vi "Target.vi"(4 "Refnums":T3, 7 "Images":T2[](array[typedef]), 8 "error in (no error)":errorcluster, 10 "Pattern Matching Criteria":T4={"Minimum Score"=700.0, "Color Score Weight"=700.0, "Minimum Contrast"=50, "Match Mode"=0, "Match Feature Mode"=0, "Subpixel Accuracy"=TRUE, "Color Sensitivity"=1, "Search Strategy"=1} {"Search Strategy" items=["Conservative", "Balance", "Aggressive", "Very Aggressive"]; "Color Sensitivity" items=["Low Sensitivity", "Medium Sensitivity", "High Sensitivity"]; "Match Feature Mode" items=["Color and Shape", "Color", "Shape"]; "Match Mode" items=["Shift Invariant", "Rotation Invariant"]}, 11 "Function":T5) -> (0 "error out":errorcluster, 2 "Target Data":T1, 3 "Target Found?":bool)   [LabVIEW 2014]
uses:
  Target Functions.ctl
  Target Refnums.ctl
  <vilib>/vision/Image Controls.llb/IMAQ Image.ctl
  <vilib>/vision/NI_Vision_Development_Module.lvlib
panel:
  out "Edge":T2(plugin-control)
  out "Image":T2(plugin-control)
  out "Template":T2(plugin-control)
  # "LICENSED MATERIALS – PROPERTY OF IBM\nCopyright IBM Corp. 2016,\nALL RIGHTS RESERVED"
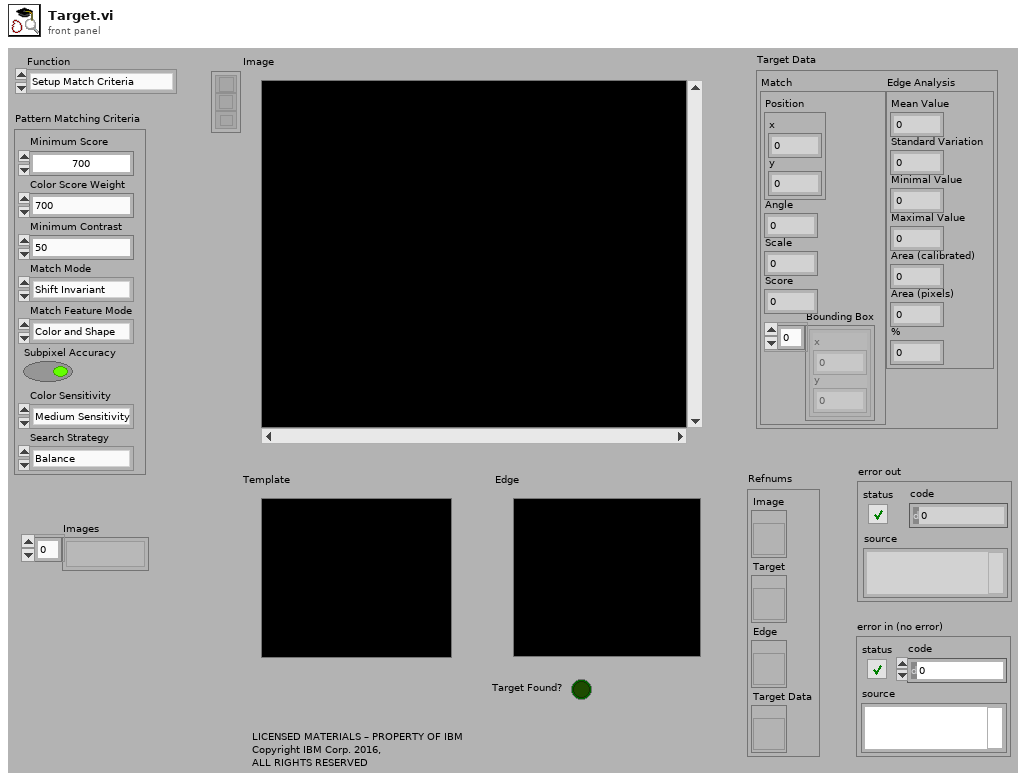
[diagram p1: front panel]
types:
  T1 = cluster{"Match":cluster{"Position":cluster{"x":sgl, "y":sgl}, "Angle":sgl, "Scale":sgl, "Score":sgl, "Bounding Box":cluster{"x":sgl, "y":sgl}[]}, "Edge Analysis":cluster{"Mean Value":sgl, "Standard Variation":sgl, "Minimal Value":sgl, "Maximal Value":sgl, "Area (calibrated)":sgl, "Area (pixels)":i32, "%":sgl}}
  T2 = typedef "IMAQ Image.ctl" = refnum<image>
  T3 = typedef "Target Refnums.ctl" = cluster{"Image":refnum<vi>, "Target":refnum<vi>, "Edge":refnum<vi>, "Target Data":refnum<vi>}
  T4 = cluster{"Minimum Score":sgl, "Color Score Weight":sgl, "Minimum Contrast":i32, "Match Mode":u32, "Match Feature Mode":u32, "Subpixel Accuracy":bool, "Color Sensitivity":u32, "Search Strategy":u32}
  T5 = typedef "Target Functions.ctl" = enum16{"Setup Match Criteria", "Set Target", "Find Target"}
  T6 = enum32{"Differentiation", "Gradient", "Prewitt", "Roberts", "Sigma", "Sobel"}
  T7 = cluster{i32[], cluster{"Contour Type":u32, "ROI Type":u32, i32[]}[]}
  T8 = cluster{"Global Rectangle":i32[], "Contours":cluster{"Contour Type":u32, "ROI Type":u32, "Points":i32[]}[]}
  T9 = cluster{"Position":cluster{"x":sgl, "y":sgl}, "Angle":sgl, "Scale":sgl, "Score":sgl, "Bounding Box":cluster{"x":sgl, "y":sgl}[]}[]
  T10 = cluster{"Position":cluster{"x":sgl, "y":sgl}, "Angle":sgl, "Scale":sgl, "Score":sgl, "Bounding Box":cluster{"x":sgl, "y":sgl}[]}
  T11 = enum8{"Enabled", "Disabled", "Disabled and Grayed Out"}
  T12 = typedef "Image Type" = u32
  T13 = cluster{"Mean Value":sgl, "Standard Variation":sgl, "Minimal Value":sgl, "Maximal Value":sgl, "Area (calibrated)":sgl, "Area (pixels)":i32, "%":sgl}
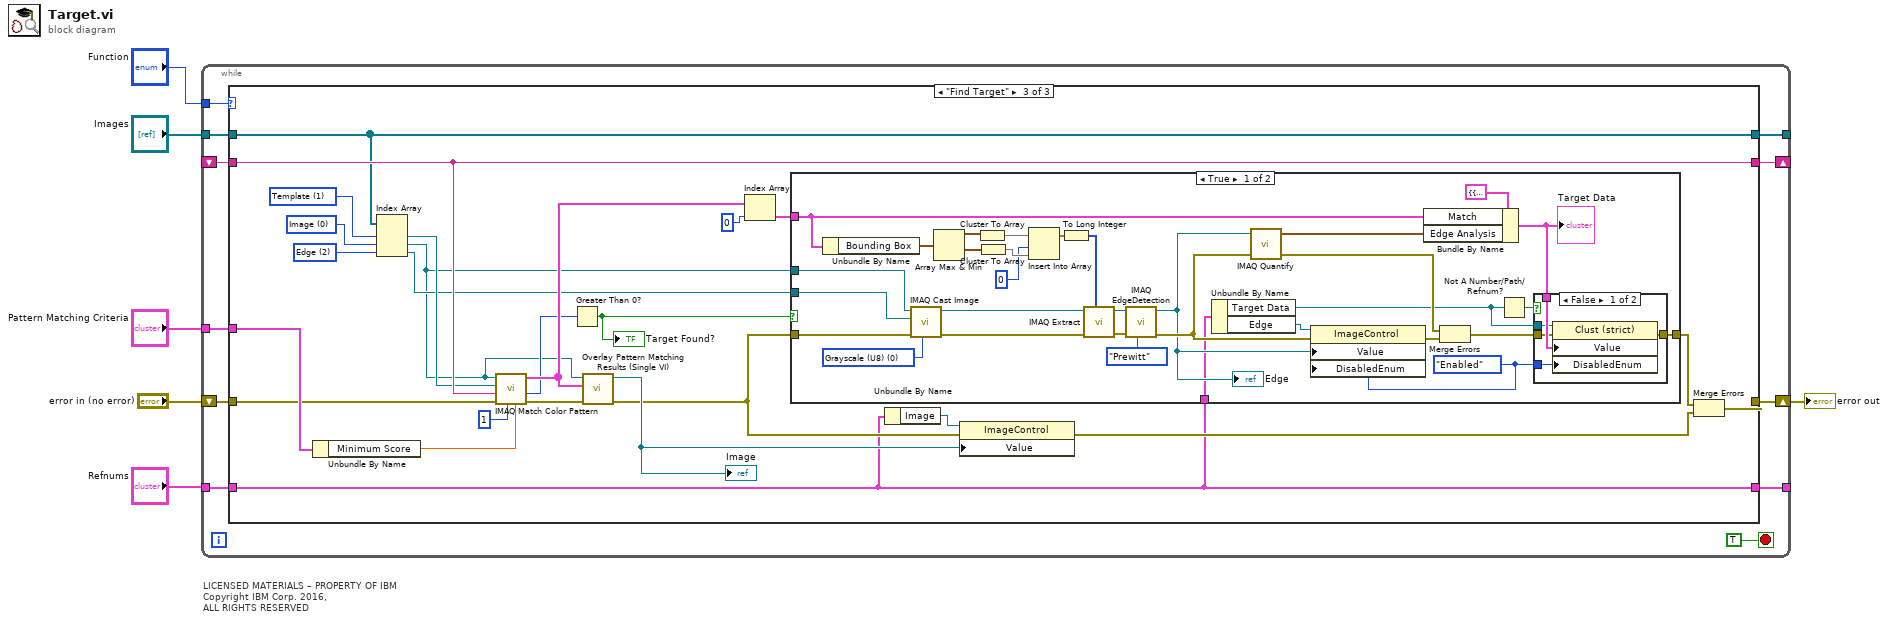
[diagram p0: block diagram]
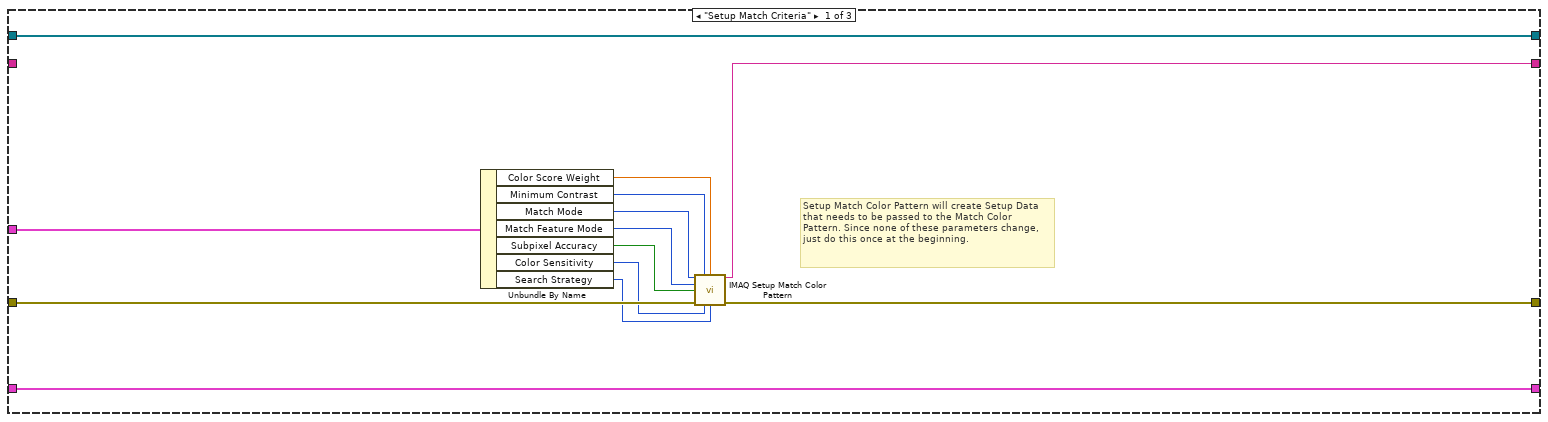
[diagram p2: hidden frame]
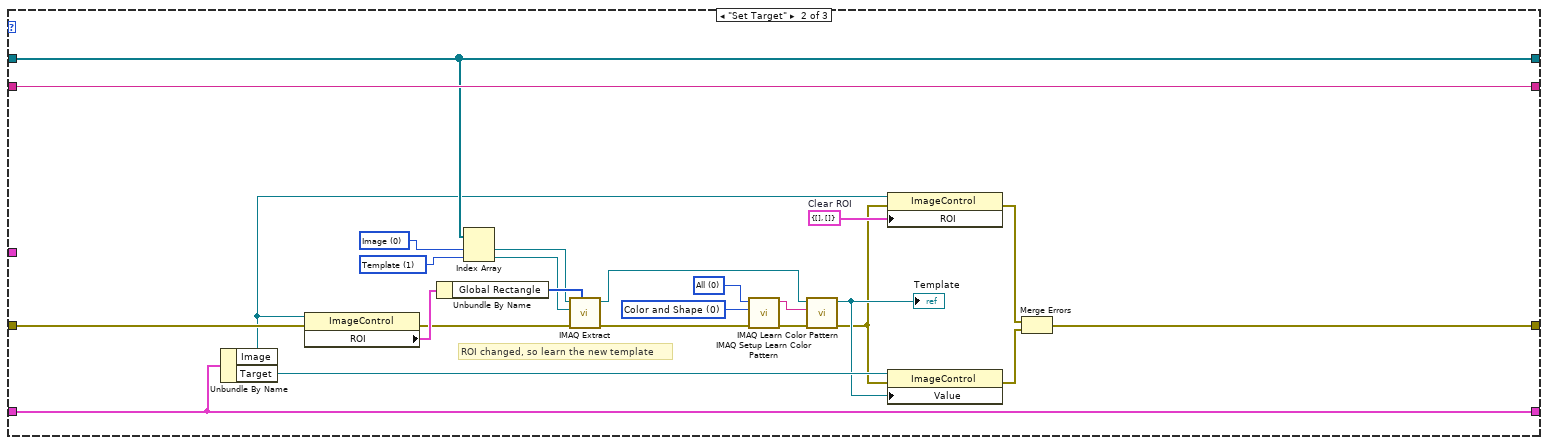
[diagram p3: hidden frame]
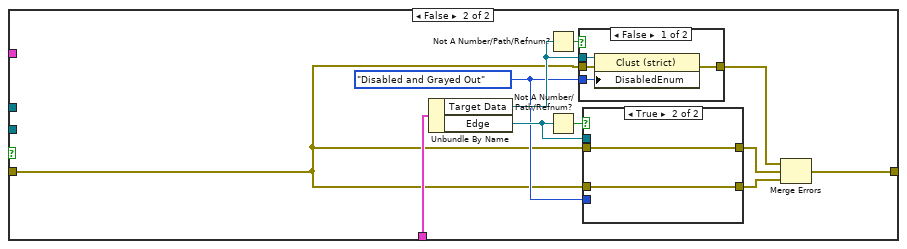
[diagram p5: hidden frame]
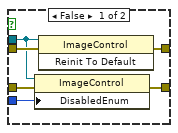
[diagram p6: hidden frame]
diagram:
  # "LICENSED MATERIALS – PROPERTY OF IBM\nCopyright IBM Corp. 2016,\nALL RIGHTS RESERVED"
  n1 = while {
    tunnel: "Function" -> [w17]
    shift-right: [w15] -> w3
    shift-left: "error in (no error)" -> [w16]
    shift-right: [w14] -> _
    shift-left: _ -> [w13]
    tunnel: "Images" -> [w12]
    tunnel: [w11] -> _
    tunnel: "Refnums" -> [w9]
    tunnel: [w10] -> _
    tunnel: "Pattern Matching Criteria" -> [w7]
    stop <- TRUE stop-if-true
    n2 = case shown="\"Find Target\"" w17 {
      tunnel: w16 -> [w30 w45 w56]
      tunnel: [w29 w32 w64] -> w15
      tunnel: [w28 w43 w76] -> w14
      tunnel: w13 -> [_ w43 w76]
      tunnel: w12 -> [w27 w42 w75]
      tunnel: [w27 w42 w75] -> w11
      tunnel: [w19 w37 w62] -> w10
      tunnel: w9 -> [w19 w37 w62]
      tunnel: w7 -> [w18 _ w58]
      frame "Setup Match Criteria" {
        # "Setup Match Color Pattern will create Setup Data that needs to be passed to the Match Color Pattern. Since none of these parameters change, just do this once at the beginning."
        n3 = Unbundle By Name(w18) -> ("Color Score Weight"=w26:sgl, "Minimum Contrast"=w25:i32, "Match Mode"=w24:u32, "Match Feature Mode"=w23:u32, "Subpixel Accuracy"=w22:bool, "Color Sensitivity"=w21:u32, "Search Strategy"=w20:u32)
        n4 = call "IMAQ Setup Match Color Pattern"("Match Mode"=w24, "Minimum Contrast"=w25, "Color Score Weight"=w26, "Match Feature Mode"=w23, "Subpixel Accuracy"=w22, "error in (no error)"=w30, "Color Sensitivity"=w21, "Search Strategy"=w20) -> ("Match Color Pattern Setup Data"=w28:string, "error out"=w29:errorcluster)  [unwired: 6 in]
      }
      frame "Set Target" {
        w40 = u16 1 items=["Image", "Template"] ("Image Names")
        w41 = u16 0 items=["Image", "Template"] ("Image Names")
        w47 = u32 0 items=["Color and Shape", "Color", "Shape "] ("Feature Mode")
        w48 = u32 0 items=["All", "Shift Information", "Rotation Information"] ("Learn Mode")
        w49 = T7 {[], []}  # Clear ROI
        # "ROI changed, so learn the new template"
        n5 = Unbundle By Name(w37) -> ("Image"=w36:refnum<vi>, "Target"=w35:refnum<vi>)
        n6 = property on="Property Node" class="ImageControl"(reference=w36, error in=w45) -> (error out=w44:errorcluster, "ROI"=w50:T8)  [unwired: 1 out]
        n7 = Unbundle By Name(w50) -> ("Global Rectangle"=w55:i32[])
        n8 = Index Array(array=w42, index #1=w41, index #2=w40) -> (element #1=w38:T2, element #2=w39:T2)
        n9 = call "IMAQ Extract"("Optional Rectangle"=w55, "error in (no error)"=w44, "Image Dst"=w39, "Image Src"=w38) -> ("error out"=w52:errorcluster, "Image Dst Out"=w53:T2)  [unwired: 6 in]
        n10 = call "IMAQ Setup Learn Color Pattern"("error in (no error)"=w52, "Feature Mode"=w47, "Learn Mode"=w48) -> ("error out"=w51:errorcluster, "Learn Color Pattern Setup Data"=w54:string)  [unwired: 7 in]
        n11 = call "IMAQ Learn Color Pattern"("error in (no error)"=w51, "Learn Color Pattern Setup Data"=w54, "Image"=w53) -> ("error out"=w33:errorcluster, "Template Image Out"=w34:T2)  [unwired: 7 in]
        "Template" <- w34
        n12 = property on="Property Node" class="ImageControl"(reference=w36, error in=w33, "ROI"=w49) -> (error out=w46:errorcluster)  [unwired: 1 out]
        n13 = property on="Property Node" class="ImageControl"(reference=w35, error in=w33, "Value"=w34) -> (error out=w31:errorcluster)  [unwired: 1 out]
        n14 = Merge Errors(w46, w31) -> (w32:errorcluster)
      }
      frame "Find Target" {
        w70 = u16 1 items=["Image", "Template", "Edge"] ("Image Names")
        w69 = u16 0 items=["Image", "Template", "Edge"] ("Image Names")
        w68 = u16 2 items=["Image", "Template", "Edge"] ("Image Names")
        n15 = Unbundle By Name(w58) -> ("Minimum Score"=w59:sgl)
        n16 = Index Array(array=w75, index #1=w70, index #2=w69, index #3=w68) -> (element #1=w74:T2, element #2=w57:T2, element #3=w60:T2)
        n17 = call "IMAQ Match Color Pattern"("Minimum Match Score"=w59, "Number of Matches Requested"=1 ("Max # of Matches"), "error in (no error)"=w56, "Match Color Pattern Setup Data"=w76, "Template Image"=w74, "Image"=w57) -> ("error out"=w80:errorcluster, "Number of Matches"=w71:i32, "Matches"=w73:T9)  [unwired: 3 in]
        n18 = Greater Than 0?(x=w71) -> (x > 0?=w61:bool)
        "Target Found?" <- w61
        n19 = call "Overlay Pattern Matching Results (Single VI).vi"("error in"=w80, "Matches"=w73, "Image"=w57) -> ("error out"=w66:errorcluster, "Image Out"=w78:T2)  [unwired: 7 in]
        "Image" <- w78
        n20 = Index Array(array=w73, index=0) -> (element=w67:T10)
        n21 = case shown="True" w61 {
          tunnel: w67 -> [w90 _]
          tunnel: w66 -> [w94 w120]
          tunnel: [w87 w123] -> w65
          tunnel: w62 -> [w92 w129]
          tunnel: w57 -> [w85 _]
          tunnel: w60 -> [w84 _]
          frame True {
            w81 = T11."Enabled" ("Disabled")
            w101 = T12 0 items=["Grayscale (U8)", "Grayscale (I16)", "Grayscale (SGL)", "Complex (CSG)", "RGB (U32)", "HSL (U32)", "RGB (U64)", "Grayscale (U16)"] ("Image Type")
            n22 = Unbundle By Name(w90) -> ("Bounding Box"=w111:cluster{"x":sgl, "y":sgl}[])
            n23 = call "IMAQ Cast Image"("Image Type"=w101, "error in (no error)"=w94, "Image Dst"=w84, "Image Src"=w85) -> ("error out"=w99:errorcluster, "Image Dst Out"=w100:T2)  [unwired: 2 in, 4 out]
            n24 = Array Max & Min(array=w111) -> (max value=w109:cluster{"x":sgl, "y":sgl}, min value=w110:cluster{"x":sgl, "y":sgl})  [unwired: 2 out]
            n25 = Cluster To Array(cluster=w109) -> (array=w108:sgl[])
            n26 = Cluster To Array(cluster=w110) -> (array=w107:sgl[])
            n27 = Insert Into Array(array=w108, index=0, new element=w107) -> (w112:sgl[])
            n28 = To Long Integer(number=w112) -> (32bit integer=w102:i32[])
            n29 = call "IMAQ Extract"("Optional Rectangle"=w102, "error in (no error)"=w99, "Image Src"=w100) -> ("error out"=w104:errorcluster, "Image Dst Out"=w103:T2)  [unwired: 3 in, 4 out]
            n30 = call "IMAQ EdgeDetection"("Method"=T6."Prewitt", "error in (no error)"=w104, "Image Src"=w103) -> ("error out"=w97:errorcluster, "Image Dst Out"=w95:T2)  [unwired: 3 in, 4 out]
            "Edge" <- w95
            n31 = Unbundle By Name(w92) -> ("Target Data"=w82:refnum<vi>, "Edge"=w93:refnum<vi>)
            n32 = call "IMAQ Quantify"("error in (no error)"=w97, "Image"=w95) -> ("error out"=w96:errorcluster, "Global Report"=w89:T13)  [unwired: 1 in, 1 out]
            n33 = property class="ImageControl"(reference=w93, error in=w97, "Value"=w95, "DisabledEnum"=w81) -> (error out=w98:errorcluster)  [unwired: 1 out]
            n34 = Bundle By Name(cluster=T1 {"Match"={"Position"={"x"=0.0, "y"=0.0}, "Angle"=0.0, "Scale"=0.0, "Score"=0.0, "Bounding Box"=[]}, "Edge Analysis"={"Mean Value"=0.0, "Standard Variation"=0.0, "Minimal Value"=0.0, "Maximal Value"=0.0, "Area (calibrated)"=0.0, "Area (pixels)"=0, "%"=0.0}} ("Target Data 2"), "Match"=w90, "Edge Analysis"=w89) -> (w88:T1)
            "Target Data" <- w88
            n35 = Merge Errors(w96, w98) -> (w86:errorcluster)
            n36 = Not A Number/Path/Refnum?(number/path/refnum=w82) -> (NaN/Path/Refnum?=w83:bool)
            n37 = case shown="False" w83 {
              tunnel: w81 -> [w117 _]
              tunnel: w88 -> [w116 _]
              tunnel: [w115 w118] -> w87
              tunnel: w86 -> [w114 w118]
              tunnel: w82 -> [w113 _]
              frame False {
                n38 = property class="Clust (strict)"(reference=w113, error in=w114, "Value"=w116, "DisabledEnum"=w117) -> (error out=w115:errorcluster)  [unwired: 1 out]
              }
              frame True {
              }
            }
          }
          frame False {
            w121 = T11."Disabled and Grayed Out" ("Disabled")
            n39 = Unbundle By Name(w129) -> ("Target Data"=w126:refnum<vi>, "Edge"=w124:refnum<vi>)
            n40 = Not A Number/Path/Refnum?(number/path/refnum=w126) -> (NaN/Path/Refnum?=w127:bool)
            n41 = Not A Number/Path/Refnum?(number/path/refnum=w124) -> (NaN/Path/Refnum?=w125:bool)
            n42 = case shown="False" w127 {
              tunnel: w121 -> [w141 _]
              tunnel: [w140 w142] -> w128
              tunnel: w126 -> [w139 _]
              tunnel: w120 -> [w138 w142]
              frame False {
                n43 = property class="Clust (strict)"(reference=w139, error in=w138, "DisabledEnum"=w141) -> (error out=w140:errorcluster)  [unwired: 1 out]
              }
              frame True {
              }
            }
            n44 = case shown="True" w125 {
              tunnel: w124 -> [w133 _]
              tunnel: w120 -> [w135 w137]
              tunnel: [w134 w137] -> w122
              tunnel: w121 -> [w132 _]
              tunnel: w120 -> [w131 w136]
              tunnel: [w130 w136] -> w119
              frame False {
                n45 = property class="ImageControl"(reference=w133, error in=w131, "DisabledEnum"=w132) -> (error out=w130:errorcluster)  [unwired: 1 out]
                n46 = invoke class="ImageControl" method="Reinit To Default"(reference=w133, error in=w135) -> (error out=w134:errorcluster)  [unwired: 1 in, 2 out]
              }
              frame True {
              }
            }
            n47 = Merge Errors(w128, w122, w119) -> (w123:errorcluster)
          }
        }
        n48 = Unbundle By Name(w62) -> ("Image"=w77:refnum<vi>)
        n49 = property class="ImageControl"(reference=w77, error in=w66, "Value"=w78) -> (error out=w63:errorcluster)  [unwired: 1 out]
        n50 = Merge Errors(w65, w63) -> (w64:errorcluster)
      }
    }
  }
  "error out" <- w3
